vi "Rotate2DArray.vi"(9 "Rot Reference":enum16{"Row Wise", "Column Wise"}(ring), 10 "Rot Index":i32, 11 "Array in":dbl[][](array[numeric])) -> (3 "Array out":dbl[][](array[numeric]))   [LabVIEW 2019]
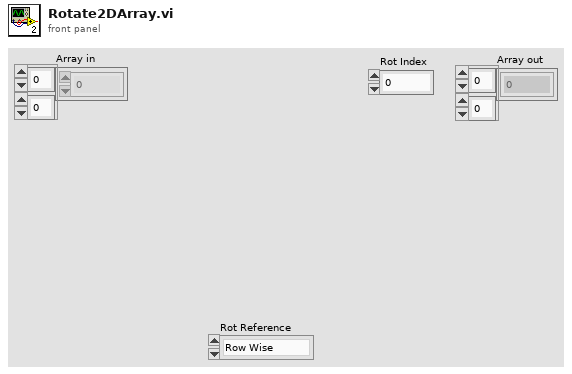
[diagram p1: front panel]
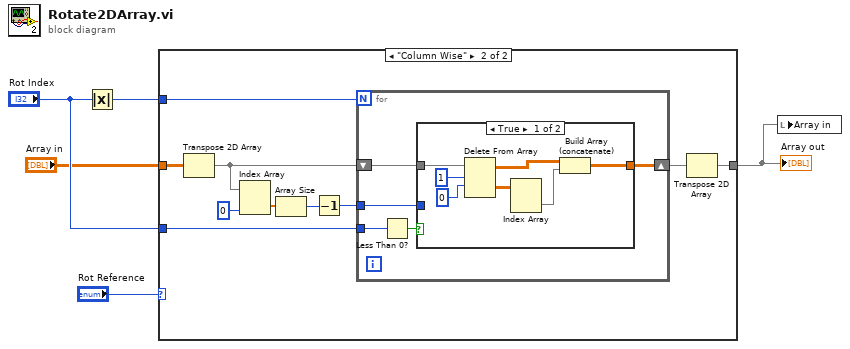
[diagram p0: block diagram]
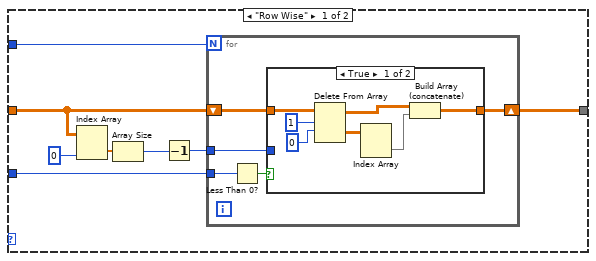
[diagram p2: hidden frame]
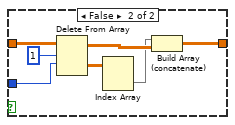
[diagram p3: hidden frame]
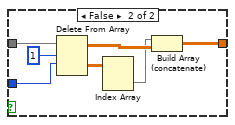
[diagram p4: hidden frame]
diagram:
  n1 = Absolute Value(x="Rot Index") -> (abs(x)=w5:i32)
  n2 = case shown="\"Column Wise\"" "Rot Reference" {
    tunnel: w5 -> [w13 w42]
    tunnel: "Array in" -> [w12 w41]
    tunnel: "Rot Index" -> [w7 w36]
    tunnel: [w6 w33] -> w2
    frame "Row Wise" {
      n3 = Index Array(array=w12, index (col)=0 ("disabled index (col)")) -> (element=w10:dbl[])  [unwired: 1 in]
      n4 = Array Size(array=w10) -> (size(s)=w8:i32)
      n5 = Decrement(x=w8) -> (x-1=w9:i32)
      n6 = for {
        N: w13 -> [_]
        shift-right: [w17] -> w6
        shift-left: w12 -> [w18]
        tunnel: w9 -> [w15]
        tunnel: w7 -> [w14]
        n7 = Less Than 0?(x=w14) -> (x < 0?=w16:bool)
        n8 = case shown="True" w16 {
          tunnel: w18 -> [w25 w32]
          tunnel: [w22 w29] -> w17
          tunnel: w15 -> [_ w27]
          frame True {
            n9 = Delete From Array(array=w25, length=1, index (row)=0) -> (deleted portion=w21:dbl[][], array with subset deleted=w24:dbl[][])  [unwired: 1 in]
            n10 = Index Array(array=w21) -> (element=w20:dbl[])  [unwired: 2 in]
            n11 = Build Array (concatenate)(w24, w20) -> (w22:dbl[][])
          }
          frame False {
            n12 = Delete From Array(array=w32, length=1, index (row)=w27) -> (deleted portion=w28:dbl[][], array with subset deleted=w31:dbl[][])  [unwired: 1 in]
            n13 = Index Array(array=w28) -> (element=w26:dbl[])  [unwired: 2 in]
            n14 = Build Array (concatenate)(w26, w31) -> (w29:dbl[][])
          }
        }
      }
    }
    frame "Column Wise" {
      n15 = Transpose 2D Array(2D array=w41) -> (transposed array=w34:dbl[][])
      n16 = Index Array(array=w34, index (col)=0 ("disabled index (col)")) -> (element=w39:dbl[])  [unwired: 1 in]
      n17 = Array Size(array=w39) -> (size(s)=w37:i32)
      n18 = Decrement(x=w37) -> (x-1=w38:i32)
      n19 = for {
        N: w42 -> [_]
        shift-right: [w46] -> w35
        shift-left: w34 -> [w47]
        tunnel: w38 -> [w44]
        tunnel: w36 -> [w43]
        n20 = Less Than 0?(x=w43) -> (x < 0?=w45:bool)
        n21 = case shown="True" w45 {
          tunnel: w47 -> [w54 w61]
          tunnel: [w51 w58] -> w46
          tunnel: w44 -> [_ w56]
          frame True {
            n22 = Delete From Array(array=w54, length=1, index (row)=0) -> (deleted portion=w50:dbl[][], array with subset deleted=w53:dbl[][])  [unwired: 1 in]
            n23 = Index Array(array=w50) -> (element=w49:dbl[])  [unwired: 2 in]
            n24 = Build Array (concatenate)(w53, w49) -> (w51:dbl[][])
          }
          frame False {
            n25 = Delete From Array(array=w61, length=1, index (row)=w56) -> (deleted portion=w57:dbl[][], array with subset deleted=w60:dbl[][])  [unwired: 1 in]
            n26 = Index Array(array=w57) -> (element=w55:dbl[])  [unwired: 2 in]
            n27 = Build Array (concatenate)(w55, w60) -> (w58:dbl[][])
          }
        }
      }
      n28 = Transpose 2D Array(2D array=w35) -> (transposed array=w33:dbl[][])
    }
  }
  "Array out" <- w2
  n29 = local write "Array in"(w2) -> ()
